vi "last_intersection_check.vi"(7 "Last intersection color":T1, 10 "Identify Color":dbl, 11 "Old color":dbl) -> (0 "Identify Color 3":dbl, 1 "Identify Color 2":dbl)   [LabVIEW 2016]
uses:
  <vilib>/NXT/Subs/ColorSensorColors.ctl
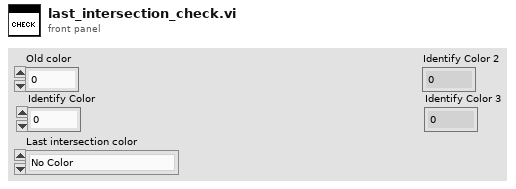
[diagram p1: front panel]
types:
  T1 = typedef "ColorSensorColors.ctl" = enum16{"No Color", "Black", "Blue", "Green", "Yellow", "Red", "White", "Brown"}
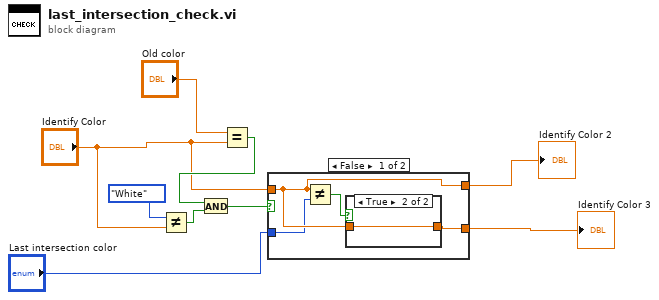
[diagram p0: block diagram]
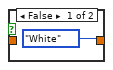
[diagram p2: hidden frame]
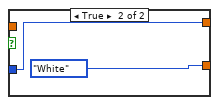
[diagram p3: hidden frame]
diagram:
  n1 = Not Equal?(x=ColorSensorColors."White", y="Identify Color") -> (x != y?=w9:bool)
  n2 = Equal?(x="Old color", y="Identify Color") -> (x = y?=w6:bool)
  n3 = And(x=w6, y=w9) -> (x .and. y?=w7:bool)
  n4 = case shown="False" w7 {
    tunnel: [w12 ColorSensorColors."White" ("Detected Color")] -> w2
    tunnel: "Identify Color" -> [w11 _]
    tunnel: [w11 w16] -> w3
    tunnel: "Last intersection color" -> [w10 w16]
    frame False {
      n5 = Not Equal?(x=w11, y=w10) -> (x != y?=w13:bool)
      n6 = case shown="True" w13 {
        tunnel: [ColorSensorColors."White" ("Detected Color") w15] -> w12
        tunnel: w11 -> [_ w15]
        frame False {
        }
        frame True {
        }
      }
    }
    frame True {
    }
  }
  "Identify Color 2" <- w3
  "Identify Color 3" <- w2
